vi "MPXgetsettings.vi"(5 "VISA resource name":refnum<visa-resource-name>="COM5") -> (0 "Signal On":bool, 1 "Amplitude [V]":i32=200 min=5 max=250 step=1, 2 "Frequence [Hz]":i32=150 min=0 max=300 step=1, 3 "Waveform":u16(ring) items=["Sine", "Rectangle", "SRS-Signal"], 4 "read buffer":string="F110\r\nFrequence changed\r\n\r\nWavetype: Triangle\r\nFrequence: 0110 Hz\r\nAmplitude: 200,0 V\r\nSignal off\r\n\r\nempc>:\n")   [LabVIEW 2015]
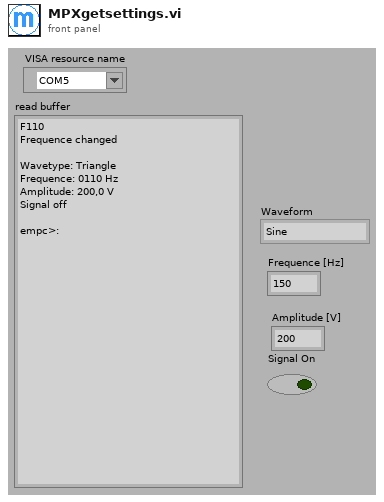
[diagram p1: front panel]
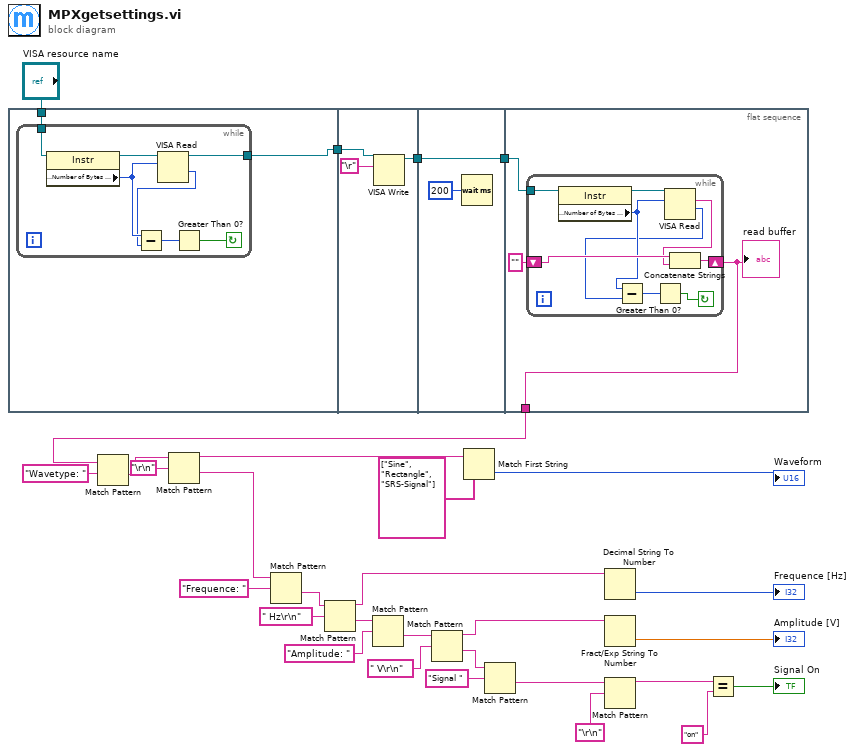
[diagram p0: block diagram]
diagram:
  n1 = flat-sequence {
    tunnel: "VISA resource name" -> [w32]
    tunnel: [w31] -> w30
    tunnel: [w41] -> w29
    tunnel: w30 -> [w40]
    tunnel: w29 -> [w44]
    tunnel: [w44] -> w28
    tunnel: w28 -> [w46]
    tunnel: [w45] -> w5
    frame #0 {
      n2 = while {
        tunnel: w32 -> [w35]
        tunnel: [w34] -> w31
        stop <- w38 continue-if-true
        n3 = property class="Instr"(reference=w35) -> (reference out=w39:refnum<visa-resource-name>, "Serial Settings:Number of Bytes at Serial Port"=w37:u32)  [unwired: 1 in, 1 out]
        n4 = VISA Read(VISA resource name=w39, byte count=w37) -> (VISA resource name out=w34:refnum<visa-resource-name>, return count=w36:u32)  [unwired: 1 in, 2 out]
        n5 = Subtract(x=w37, y=w36) -> (x-y=w33:u32)
        n6 = Greater Than 0?(x=w33) -> (x > 0?=w38:bool)
      }
    }
    frame #1 {
      n7 = VISA Write(VISA resource name=w40, write buffer="\r") -> (VISA resource name out=w41:refnum<visa-resource-name>)  [unwired: 1 in, 2 out]
    }
    frame #2 {
      n8 = Wait (ms)(milliseconds to wait=u32 200) -> ()  [unwired: 1 out]
    }
    frame #3 {
      n9 = while {
        tunnel: w46 -> [w55]
        shift-right: [w53] -> w45
        shift-left: "" -> [w54]
        stop <- w48 continue-if-true
        n10 = property class="Instr"(reference=w55) -> (reference out=w56:refnum<visa-resource-name>, "Serial Settings:Number of Bytes at Serial Port"=w50:u32)  [unwired: 1 in, 1 out]
        n11 = VISA Read(VISA resource name=w56, byte count=w50) -> (read buffer=w52:string, return count=w49:u32)  [unwired: 1 in, 2 out]
        n12 = Subtract(x=w50, y=w49) -> (x-y=w51:u32)
        n13 = Greater Than 0?(x=w51) -> (x > 0?=w48:bool)
        n14 = Concatenate Strings(w54, w52) -> (w53:string)
      }
      "read buffer" <- w45
    }
  }
  n15 = Match Pattern(string=w5, regular expression="Wavetype: " ("search string/char (-)")) -> (after substring=w21:string)  [unwired: 1 in, 3 out]
  n16 = Match Pattern(string=w21, regular expression="\r\n") -> (before substring=w19:string, after substring=w23:string)  [unwired: 1 in, 2 out]
  n17 = Match Pattern(string=w23, regular expression="Frequence: ") -> (after substring=w20:string)  [unwired: 1 in, 3 out]
  n18 = Match Pattern(string=w20, regular expression=" Hz\r\n") -> (before substring=w17:string, after substring=w13:string)  [unwired: 1 in, 2 out]
  n19 = Match Pattern(string=w13, regular expression="Amplitude: ") -> (after substring=w16:string)  [unwired: 1 in, 3 out]
  n20 = Match Pattern(string=w16, regular expression=" V\r\n") -> (before substring=w12:string, after substring=w8:string)  [unwired: 1 in, 2 out]
  n21 = Match First String(2:string[] ["Sine", "Rectangle", "SRS-Signal"] ("string array"), 3:w19) -> (0:→"Waveform":i32)  [unwired: 1 out]
  n22 = Match Pattern(string=w8, regular expression="Signal ") -> (after substring=w9:string)  [unwired: 1 in, 3 out]
  n23 = Decimal String To Number(string=w17) -> (number=→"Frequence [Hz]":i32)  [unwired: 2 in, 1 out]
  n24 = Fract/Exp String To Number(string=w12) -> (number=→"Amplitude [V]":dbl)  [unwired: 3 in, 1 out]
  n25 = Match Pattern(string=w9, regular expression="\r\n") -> (before substring=w7:string)  [unwired: 1 in, 3 out]
  n26 = Equal?(x=w7, y="on") -> (x = y?=→"Signal On":bool)
